vi "THDG.vi"(8 "error in (no error)":errorcluster, 9 "system info in":refnum<class "EP System Info.lvclass">, 11 "harmonic groups complex spectra":cluster{"f0":dbl, "df":dbl, "vectors":cdb[]}[](array[cluster])) -> (0 "error out":errorcluster, 1 "system info out":refnum<class "EP System Info.lvclass">, 3 "THDG [%]":dbl[](array[numeric]))   [LabVIEW 2014, in "NI_EP_Power Quality.lvlib"]
doc: "Calculates group total harmonic distortion and subgroup total harmonic distortion, in percentage, according to IEC 61000-4-7:2009. You must manually select the polymorphic instance to use.\n\nThis VI supports measuring single-line and multiple-line systems."
uses:
  <vilib>/addons/Electrical Power/PQ/NI_EP_Power Quality.lvlib
  <vilib>/addons/Electrical Power/PQ/Common/Classes/System Info/EP System Info.lvclass
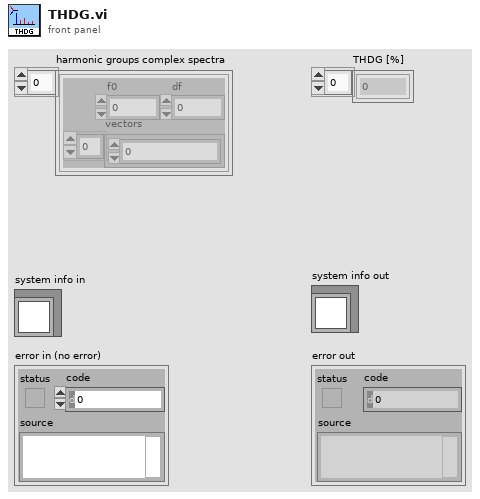
[diagram p1: front panel]
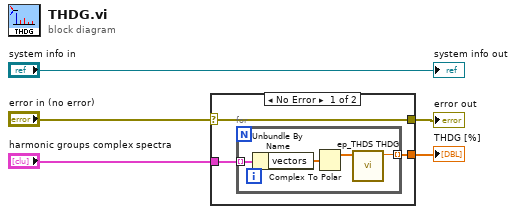
[diagram p0: block diagram]
diagram:
  n1 = case shown="No Error" "error in (no error)" {
    selector: "error in (no error)" -> [w6 w13]
    tunnel: "harmonic groups complex spectra" -> [w8 _]
    tunnel: [w7 _] -> w2
    tunnel: [w6 w13] -> w1
    frame No Error {
      n2 = for {
        tunnel: w8 -> [w12] mode=indexing
        tunnel: [w11] -> w7 mode=indexing
        n3 = Unbundle By Name(w12) -> ("vectors"=w10:cdb[])
        n4 = Complex To Polar(r * e^(i*theta)=w10) -> (r=w9:dbl[])  [unwired: 1 out]
        n5 = call <vilib>:"ep_THDS THDG.vi"("Array"=w9) -> ("Numeric"=w11:dbl)  [unwired: 10 in]
      }
    }
    frame Error {
    }
  }
  "error out" <- w1
  "THDG [%]" <- w2
  "system info out" <- "system info in"
